vi "Iterate.vi"(8 "error in (no error)":errorcluster, 10 "Iterator Settings":T1={"Prepare timeout (ms)"=200, "Iterate timeout (ms)"=50, "Conclude timeout (ms)"=200, "Iterate period (ms)"=200, "Number of iterations"=5, "Time before stop (ms)"=5, "Active Stop Conditions"={"Number of Iterations"=FALSE, "Time Elapsed"=FALSE, "Iteration Result"=FALSE}, "Prepare Msg"=refnum, "Iterate Msg"=refnum, "Conclude Msg"=refnum, "Iterations End Report"=refnum, "Message Priority (Normal)"=enum."Normal"}, 11 "Iterator Actor in":refnum<class "Iterator NR Actor.lvclass">) -> (0 "error out":errorcluster, 3 "Iterator Actor out":refnum<class "Iterator NR Actor.lvclass">)   [LabVIEW 2023, in "Iterator Actor.lvlib" / "Iterator NR Actor.lvclass"]
doc: "Iteratively calls the Iterate method of the Client. \nStops the iterations either by receiving the Stop signal, or by any of predefined Stop conditions."
uses:
  Iterator NR Actor.lvclass
  Abstract Iterator Actor/Iterator Settings.ctl
  Abstract Iterator Actor Messages/Iterator Report Iterations End Msg/Iterator Report Iterations End Msg.lvclass
  <vilib>/ActorFramework/Message/Message.lvclass
  Abstract Iterator Actor/Active Stop Conditions.ctl
  <vilib>/ActorFramework/Message Enqueuer/Message Priority.ctl
  C:/Projects/Iterator Actor/Abstract Iterator Actor/Abstract Iterator Actor.lvclass
  C:/Program Files/National Instruments/LabVIEW 2023/vi.lib/ActorFramework/Actor/Actor.lvclass
  Abstract Iterator Actor/Abstract Iterator Actor.lvclass/Abstract Iterator Actor.ctl
  Abstract Iterator Actor/Stop Reason.ctl
  <vilib>/ActorFramework/Actor/Actor.lvclass/Actor.ctl
  <vilib>/ActorFramework/Message Enqueuer/Message Enqueuer.lvclass/Message Enqueuer.ctl
  Iterator NR Actor.lvclass/Iterator NR Actor.ctl
  <vilib>/ActorFramework/Batch Msg/Batch Msg.lvclass/Batch Msg.ctl
  Abstract Iterator Actor/Read Stop Iterate Notifier.vi
  <vilib>/ActorFramework/Message Enqueuer/Init from Existing Queue.vi
  <vilib>/ActorFramework/Actor/Read Caller Enqueuer.vi
  <vilib>/ActorFramework/Batch Msg/Send Batch.vi
  <vilib>/ActorFramework/Message Enqueuer/Enqueue.vi
  Iterator NR Actor Messages/Request Iteration Notification Msg/Request Iteration Notification Msg.lvclass
  C:/Program Files/National Instruments/LabVIEW 2023/vi.lib/ActorFramework/Message/Message.lvclass
  <vilib>/ActorFramework/Batch Msg/Batch Msg.lvclass
  <userlib>/_OpenG.lib/lvdata/lvdata.llb/LVOOP Is Same Or Descendant Class__ogtk.vi
  Abstract Iterator Actor/Read Settings.vi
  <vilib>/ActorFramework/Message Priority Queue/Priority Enqueue.vi
  <vilib>/Utility/error.llb/Error Cluster From Error Code.vi
  <vilib>/ActorFramework/Message Enqueuer/Message Enqueuer.lvclass
  Iterator NR Actor Messages/Abstract Iteration Msg/Abstract Iteration Msg.lvclass
  <vilib>/ErrorRing/Error Ring.xnode
  <userlib>/_OpenG.lib/time/time.llb/openg_time.lvlib
  Abstract Iterator Actor Messages/Write Stop Reason Msg/Write Stop Reason Msg.lvclass
  <vilib>/ActorFramework/Actor/Actor.lvclass
  Abstract Iterator Actor/Abstract Iterator Actor.lvclass
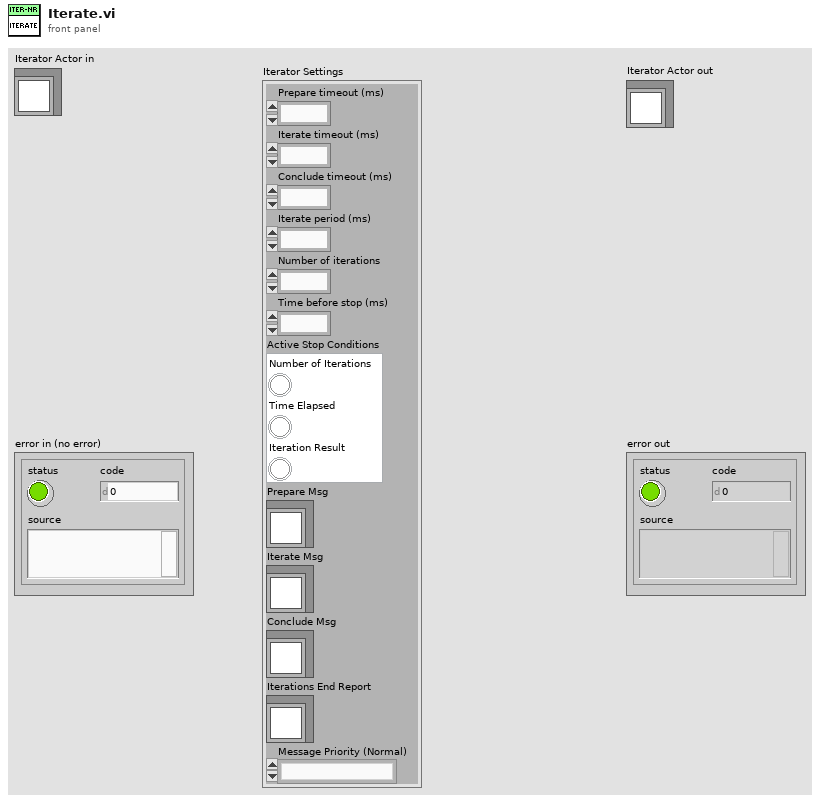
[diagram p1: front panel]
types:
  T1 = typedef "Iterator Actor.lvlib/Abstract Iterator Actor.lvclass/Iterator Settings.ctl" = cluster{"Prepare timeout (ms)":i32, "Iterate timeout (ms)":i32, "Conclude timeout (ms)":i32, "Iterate period (ms)":i32, "Number of iterations":i32, "Time before stop (ms)":i32, "Active Stop Conditions":T2, "Prepare Msg":refnum<class "Message.lvclass">, "Iterate Msg":refnum<class "Message.lvclass">, "Conclude Msg":refnum<class "Message.lvclass">, "Iterations End Report":refnum<class "Iterator Report Iterations End Msg.lvclass">, "Message Priority (Normal)":T3}
  T2 = typedef "Iterator Actor.lvlib/Abstract Iterator Actor.lvclass/Active Stop Conditions.ctl" = cluster{"Number of Iterations":bool, "Time Elapsed":bool, "Iteration Result":bool}
  T3 = typedef "Actor Framework.lvlib/Message Enqueuer.lvclass/Message Priority.ctl" = enum16{"Low", "Normal", "High"}
  T4 = typedef "Iterator Actor.lvlib/Abstract Iterator Actor.lvclass/Stop Reason.ctl" = enum16{"Number of Iterations", "Time Elapsed", "Stopped Internally", "Stopped Externally"}
  T5 = typedef "Iterator Actor.lvlib/Abstract Iterator Actor.lvclass/Stop Condition.ctl" = enum16{"None", "Number of Iterations", "Time Elapsed", "Iteration Result"}
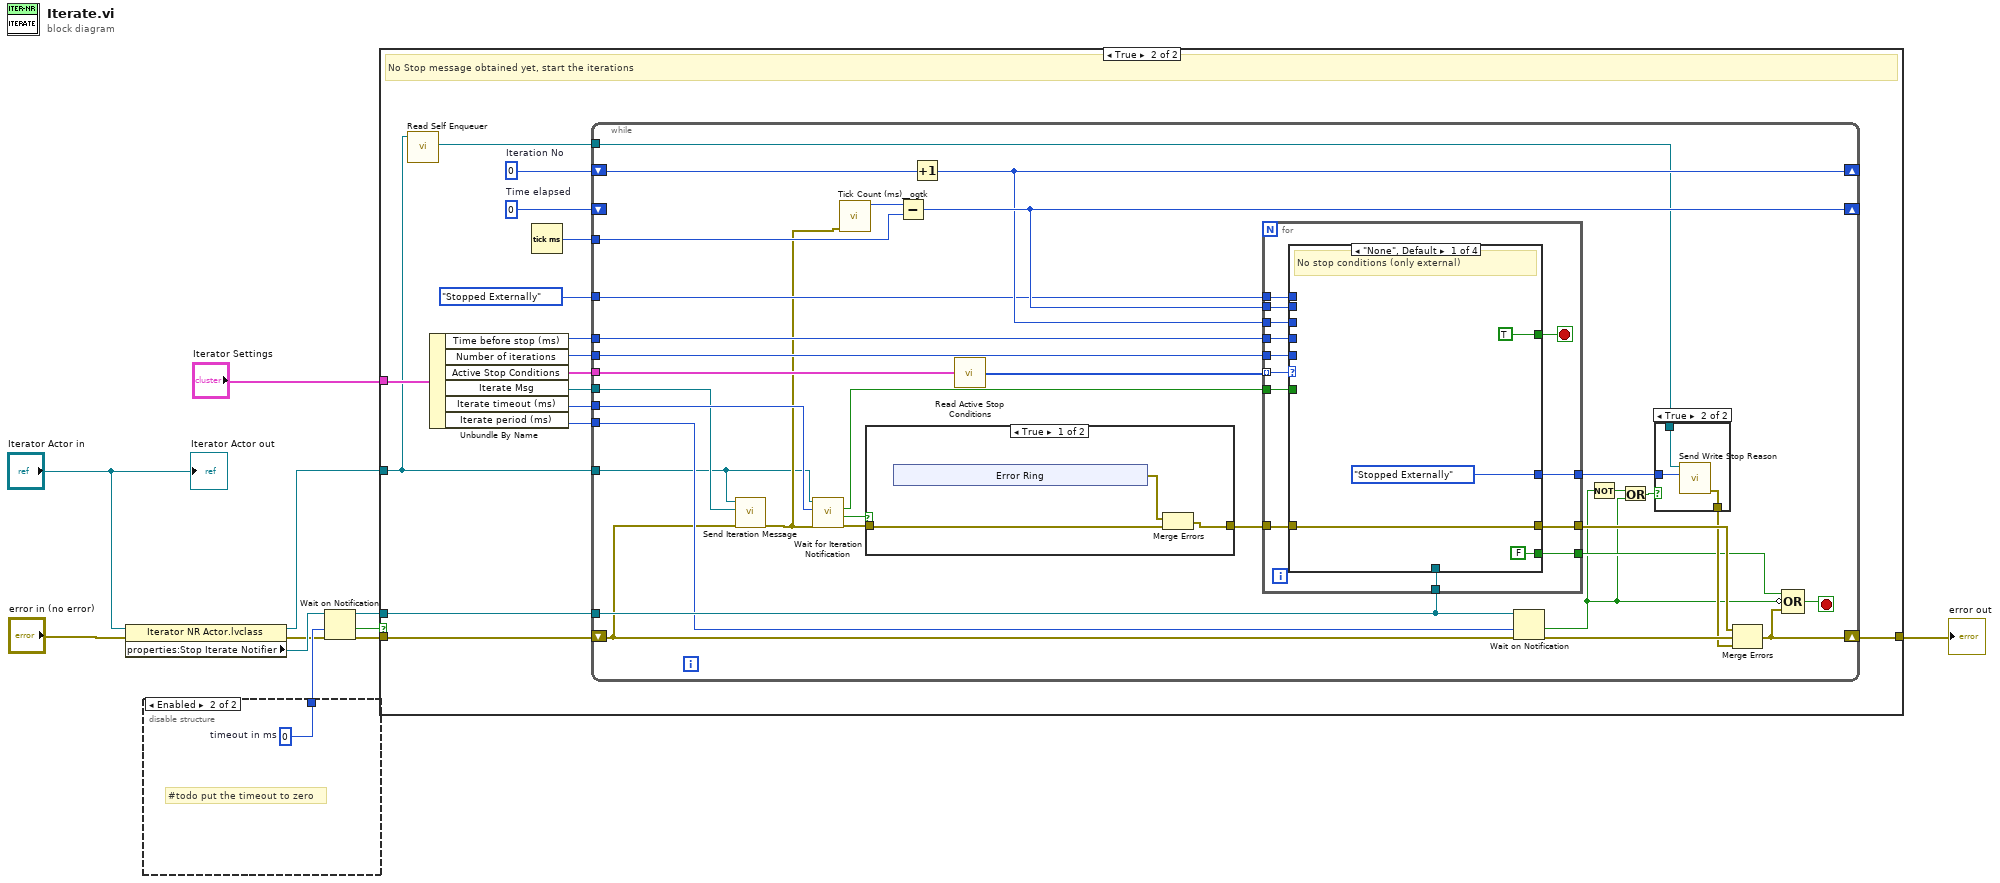
[diagram p0: block diagram]
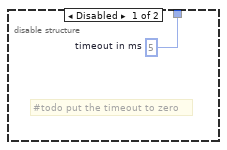
[diagram p2: hidden frame]
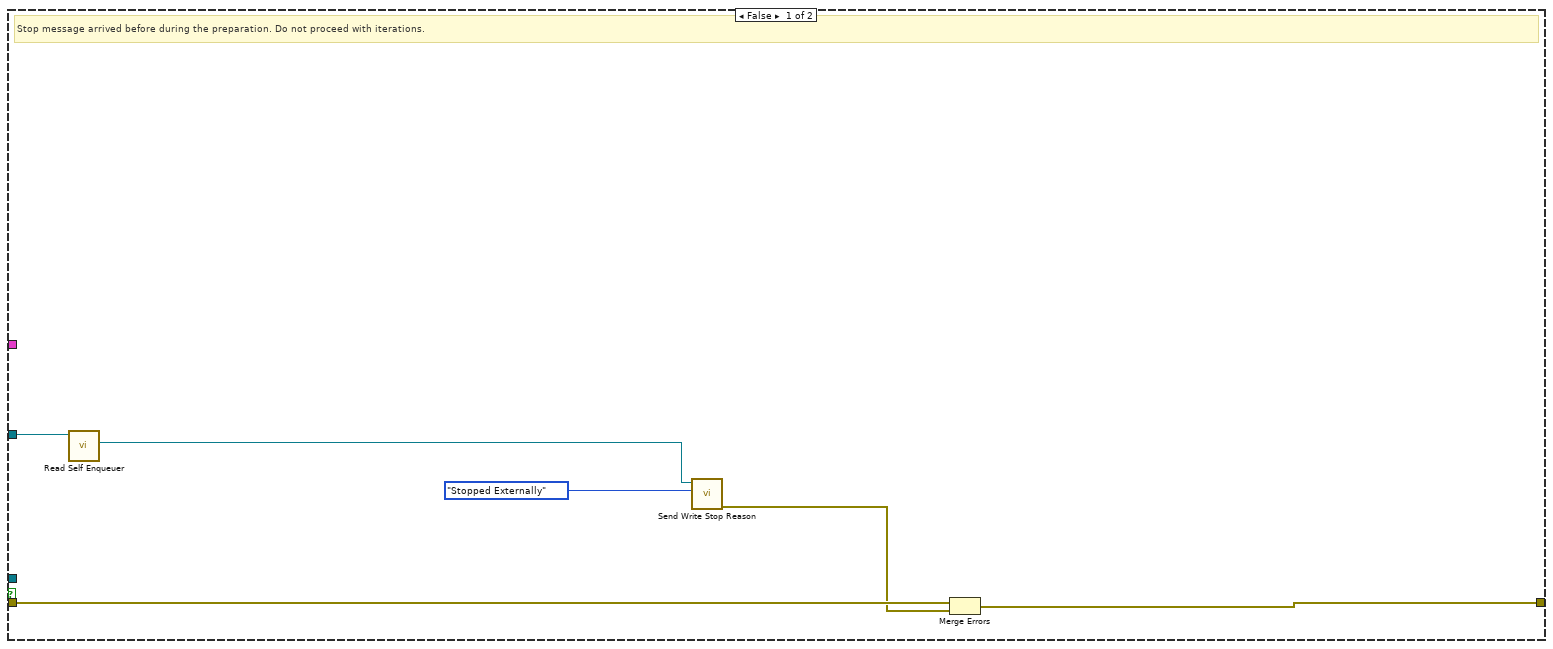
[diagram p3: hidden frame]
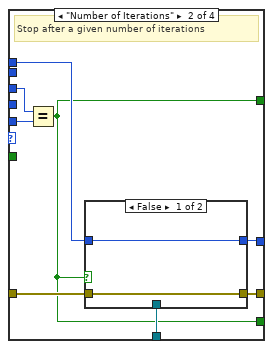
[diagram p5: hidden frame]
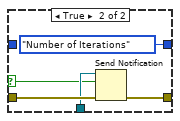
[diagram p6: hidden frame]
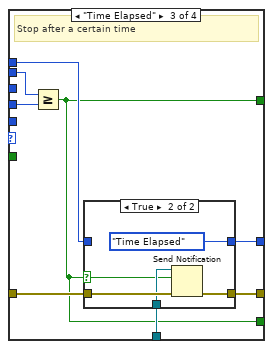
[diagram p7: hidden frame]
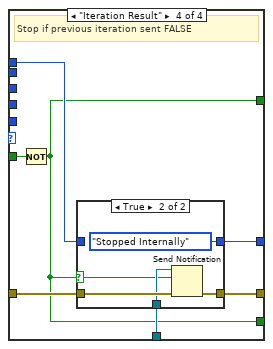
[diagram p9: hidden frame]
diagram:
  n1 = property class="Iterator NR Actor.lvclass"(reference="Iterator Actor in", error in="error in (no error)") -> (reference out=w1:refnum<class "Iterator NR Actor.lvclass">, error out=w3:errorcluster, "properties:Stop Iterate Notifier"=w5:refnum<notifier>)
  n2 = disable-structure shown="Enabled" {
    disable-tunnel: [w12 w13] -> w6
    frame Disabled {
      w12 = 5  # timeout in ms
      # "#todo put the timeout to zero"
    }
    frame Enabled {
      w13 = 0  # timeout in ms
      # "#todo put the timeout to zero"
    }
  }
  n3 = Wait on Notification(notifier=w5, timeout in ms (-1)=w6, error in (no error)=w3) -> (notifier out=w8:refnum<notifier>, timed out?=w7:bool, error out=w9:errorcluster)  [unwired: 1 in, 1 out]
  n4 = case shown="True" w7 {
    tunnel: "Iterator Settings" -> [_ w29]
    tunnel: [w17 w25] -> w10
    tunnel: w9 -> [w19 w24]
    tunnel: w8 -> [_ w23]
    tunnel: w1 -> [w15 w20]
    frame False {
      # "Stop message arrived before during the preparation. Do not proceed with iterations."
      n5 = call <vilib>:"Read Self Enqueuer.vi"("Actor"=w15) -> ("Self Enqueuer"=w14:refnum<class "Message Enqueuer.lvclass">)  [unwired: 10 in]
      n6 = call "Send Write Stop Reason.vi"("Stop Reason"=Stop_Reason."Stopped Externally", "Message Enqueuer in"=w14) -> ("error out"=w16:errorcluster)  [unwired: 8 in, 1 out]
      n7 = Merge Errors(w19, w16) -> (w17:errorcluster)
    }
    frame True {
      w26 = 0  # Iteration No
      w27 = u32 0  # Time elapsed
      # "No Stop message obtained yet, start the iterations"
      n8 = call <vilib>:"Read Self Enqueuer.vi"("Actor"=w20) -> ("Self Enqueuer"=w21:refnum<class "Message Enqueuer.lvclass">)  [unwired: 10 in]
      n9 = Unbundle By Name(w29) -> ("Time before stop (ms)"=w30:i32, "Number of iterations"=w31:i32, "Active Stop Conditions"=w32:T2, "Iterate Msg"=w33:refnum<class "Message.lvclass">, "Iterate timeout (ms)"=w34:i32, "Iterate period (ms)"=w35:i32)
      n10 = Tick Count (ms)() -> (millisecond timer value=w28:u32)
      n11 = while {
        tunnel: w33 -> [w40]
        tunnel: w34 -> [w48]
        tunnel: w35 -> [w55]
        shift-right: [w56] -> w25
        shift-left: w24 -> [w42]
        shift-right: [w58] -> _
        shift-left: w26 -> [w65]
        shift-right: [w59] -> _
        shift-left: w27 -> [_]
        tunnel: w32 -> [w50]
        tunnel: w31 -> [w64]
        tunnel: w30 -> [w63]
        tunnel: w28 -> [w60]
        tunnel: w23 -> [w57]
        tunnel: w21 -> [w54]
        tunnel: Stop_Reason."Stopped Externally" ("Stop Reason") -> [w51]
        tunnel: w20 -> [w39]
        stop <- w62 stop-if-true
        n12 = call "Send Iteration Message.vi"("error in (no error)"=w42, "Iteration Msg"=w40, "Iterator NR Actor in"=w39) -> ("error out"=w41:errorcluster)  [unwired: 8 in]
        n13 = call "Wait for Iteration Notification.vi"("error in (no error)"=w41, "timeout in ms (-1)"=w48, "Iterator NR Actor in"=w39) -> ("error out"=w38:errorcluster, "timed out?"=w37:bool, "Iterate?"=w47:bool)  [unwired: 5 in, 1 out]
        n14 = call <userlib>:"Tick Count (ms)__ogtk.vi"("error in (no error)"=w41) -> ("millisecond timer value"=w61:u32)  [unwired: 9 in, 1 out]
        n15 = case shown="True" w37 {
          tunnel: w38 -> [w70 w75]
          tunnel: [w69 w75] -> w36
          frame True {
            n16 = xnode "Error Ring"() -> ("error out"=w68:errorcluster)
            n17 = Merge Errors(w68, w70) -> (w69:errorcluster)
          }
          frame False {
          }
        }
        n18 = Subtract(x=w61, y=w60) -> (x-y=w59:u32)
        n19 = Increment(x=w65) -> (x+1=w58:i32)
        n20 = call "Read Active Stop Conditions.vi"("Active Stop Conditions"=w50) -> ("Active Stop Conditions"=w49:T5[])
        n21 = for {
          tunnel: w49 -> [w87] mode=indexing
          tunnel: w64 -> [w86]
          tunnel: w63 -> [w85]
          tunnel: w59 -> [w83]
          tunnel: w58 -> [w82]
          tunnel: w47 -> [w81]
          tunnel: w57 -> [w80]
          tunnel: w36 -> [w84]
          tunnel: [w88] -> w66
          tunnel: w51 -> [w78]
          tunnel: [w79] -> w53
          tunnel: [w76] -> w46
          stop <- w77 stop-if-true
          n22 = case shown="\"None\", Default" w87 {
            tunnel: w84 -> [w92 w98 w115 w127]
            tunnel: [w92 w97 w114 w129] -> w88
            tunnel: w80 -> [_ w100 w113 w128]
            tunnel: w86 -> [_ w99 _ _]
            tunnel: w85 -> [_ _ w112 _]
            tunnel: w83 -> [_ _ w111 _]
            tunnel: w82 -> [_ w96 _ _]
            tunnel: w81 -> [_ _ _ w124]
            tunnel: [Stop_Reason."Stopped Externally" ("Stop Reason") w95 w110 w126] -> w79
            tunnel: w78 -> [_ w94 w109 w125]
            tunnel: [TRUE ("Reply") w93 w108 w123] -> w77
            tunnel: [FALSE w93 w108 w123] -> w76
            frame "None", Default {
              # "No stop conditions (only external)"
            }
            frame "Number of Iterations" {
              # "Stop after a given number of iterations"
              n23 = Equal?(x=w96, y=w99) -> (x = y?=w93:bool)
              n24 = case shown="False" w93 {
                selector: w93 -> [_ w104]
                tunnel: w100 -> [_ w105]
                tunnel: w98 -> [w102 w107]
                tunnel: [w102 w106] -> w97
                tunnel: [w101 Stop_Reason."Number of Iterations" ("Stop Reason")] -> w95
                tunnel: w94 -> [w101 _]
                frame False {
                }
                frame True {
                  n25 = Send Notification(notification=w104, notifier=w105, error in (no error)=w107) -> (error out=w106:errorcluster)  [unwired: 1 out]
                }
              }
            }
            frame "Time Elapsed" {
              # "Stop after a certain time"
              n26 = Greater Or Equal?(x=w111, y=w112) -> (x >= y?=w108:bool)
              n27 = case shown="True" w108 {
                selector: w108 -> [_ w119]
                tunnel: w113 -> [_ w120]
                tunnel: w115 -> [w117 w122]
                tunnel: [w117 w121] -> w114
                tunnel: [w116 Stop_Reason."Time Elapsed" ("Stop Reason")] -> w110
                tunnel: w109 -> [w116 _]
                frame False {
                }
                frame True {
                  n28 = Send Notification(notification=w119, notifier=w120, error in (no error)=w122) -> (error out=w121:errorcluster)  [unwired: 1 out]
                }
              }
            }
            frame "Iteration Result" {
              # "Stop if previous iteration sent FALSE"
              n29 = Not(x=w124) -> (.not. x?=w123:bool)
              n30 = case shown="True" w123 {
                selector: w123 -> [_ w133]
                tunnel: w128 -> [_ w134]
                tunnel: w127 -> [w131 w136]
                tunnel: [w131 w135] -> w129
                tunnel: [w130 Stop_Reason."Stopped Internally" ("Stop Reason")] -> w126
                tunnel: w125 -> [w130 _]
                frame False {
                }
                frame True {
                  n31 = Send Notification(notification=w133, notifier=w134, error in (no error)=w136) -> (error out=w135:errorcluster)  [unwired: 1 out]
                }
              }
            }
          }
        }
        n32 = Wait on Notification(notifier=w57, timeout in ms (-1)=w55, error in (no error)=w42) -> (timed out?=w44:bool, error out=w67:errorcluster)  [unwired: 1 in, 2 out]
        n33 = Not(x=w44) -> (.not. x?=w43:bool)
        n34 = Or(x=w43, y=w44) -> (x .or. y?=w45:bool)
        n35 = case shown="True" w45 {
          tunnel: w54 -> [_ w139]
          tunnel: w53 -> [_ w138]
          tunnel: [_ w137] -> w52
          frame False {
          }
          frame True {
            n36 = call "Send Write Stop Reason.vi"("Stop Reason"=w138, "Message Enqueuer in"=w139) -> ("error out"=w137:errorcluster)  [unwired: 8 in, 1 out]
          }
        }
        n37 = Merge Errors(w66, w67, w52) -> (w56:errorcluster)
        n38 = Compound Arithmetic op=OR(w46, invert w44, w56) -> (w62:bool)
      }
    }
  }
  "error out" <- w10
  "Iterator Actor out" <- "Iterator Actor in"
